vi "Voltage - Continuous Input.vi"() -> ()   [LabVIEW 2018]
doc: "This example demonstrates how to continuously acquire buffered voltage measurements using a DAQmx device.\n\nFor instructions on how to connect your signals to the DAQ device, refer to your device documentation."
uses:
  <vilib>/DAQmx/read.llb/DAQmx Read (Analog 1D Wfm NChan NSamp).vi
  <vilib>/DAQmx/create/channels.llb/DAQmx Create Channel (AI-Voltage-Basic).vi
  <vilib>/DAQmx/configure/timing.llb/DAQmx Timing (Sample Clock).vi
  <vilib>/DAQmx/configure/task.llb/DAQmx Configure Logging (TDMS).vi
  <vilib>/DAQmx/configure/trigger.llb/DAQmx Start Trigger (Digital Edge).vi
  <vilib>/DAQmx/miscellaneous.llb/DAQmx Fill In Error Info.vi
  <resource>/objmgr/daqmx.rc
panel:
  in  "edge 2":i32(ring)=10280 items=["Rising"=10280, "Falling"=10171]
  in  "source 2":tag
  in  "Stop":bool
  out "Waveform Graph":waveform(dbl)[](graph)
  in  "TDMS File Path":path
  in  "Samples per Loop":i32=1000
  in  "Sample Rate":dbl=1000.0
  in  "Sample Clock Source":tag="OnboardClock"
  in  "Terminal Configuration":i32(ring)=-1 items=["default"=-1, "RSE"=10083, "NRSE"=10078, "Differential"=10106, "Pseudodifferential"=12529]
  in  "Max Voltage":dbl=5.0
  in  "Min Voltage":dbl=-5.0
  in  "Physical Channel":tag="Dev1/ai0"
  out "Actual Sample Rate":dbl=1000.0 format="%0.2f"
  in  "Logging Mode":i32(ring)=10231 items=["Off"=10231, "Log and Read"=15842]
  # "Channel Settings"
  # "Acquired Data"
  # "Timing Settings"
  # "Logging Settings"
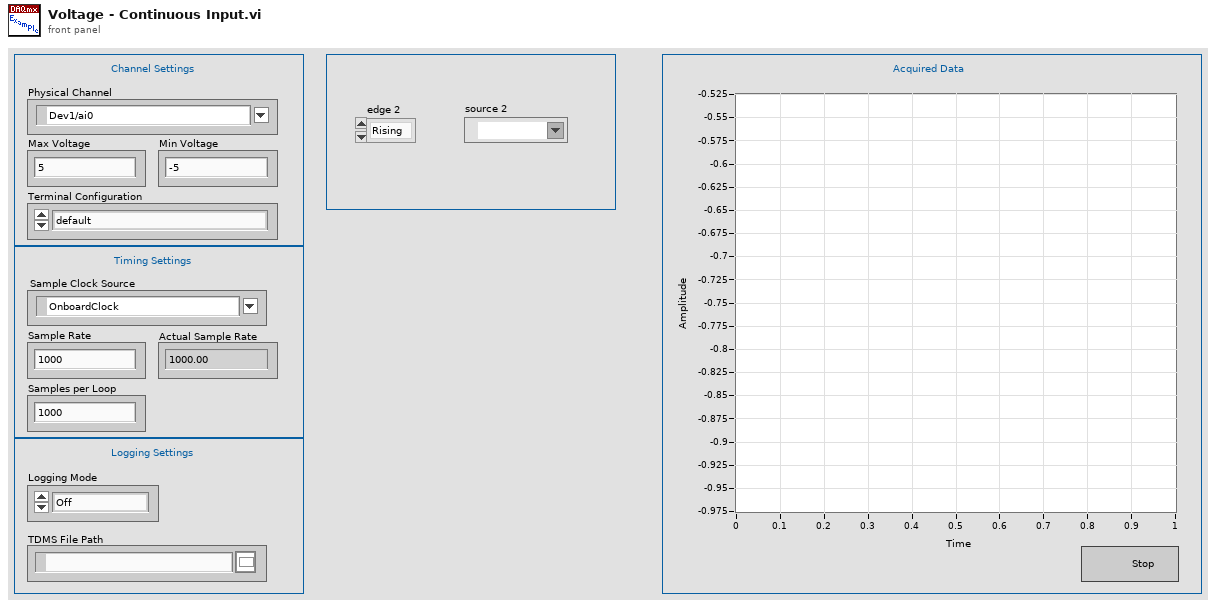
[diagram p1: front panel]
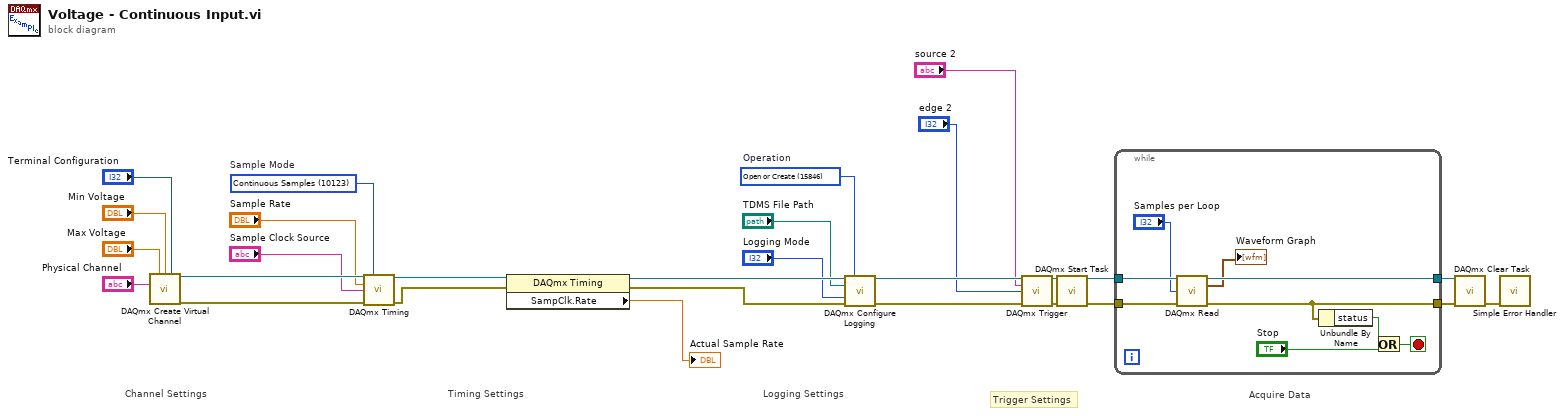
[diagram p0: block diagram]
diagram:
  w20 = 15846 items=["Open"=10437, "Open or Create"=15846, "Create or Replace"=15847, "Create"=15848]  # Operation
  w25 = 10123 items=["Finite Samples"=10178, "Continuous Samples"=10123, "Hardware Timed Single Point"=12522]  # Sample Mode
  # "Trigger Settings"
  # "Acquire Data"
  # "Timing Settings"
  # "Channel Settings"
  # "Logging Settings"
  n1 = call-poly <vilib>:"DAQmx Create Virtual Channel.vi"("maximum value"="Max Voltage", "minimum value"="Min Voltage", "input terminal configuration"="Terminal Configuration", "physical channels"="Physical Channel") -> ("task out"=w23:refnum<k21>, "error out"=w24:errorcluster)  [unwired: 10 in]
  n2 = call-poly <vilib>:"DAQmx Timing.vi"("task/channels in"=w23, "sample mode"=w25, "rate"="Sample Rate", "source"="Sample Clock Source", "error in"=w24) -> ("task out"=w27:refnum<k21>, "error out"=w26:errorcluster)  [unwired: 9 in]
  n3 = property class="DAQmx Timing"(reference=w27, error in=w26) -> (reference out=w22:refnum<k21>, error out=w21:errorcluster, "SampClk.Rate"=→"Actual Sample Rate":dbl)
  n4 = call-poly <vilib>:"DAQmx Configure Logging.vi"("task/channels in"=w22, "operation"=w20, "file path"="TDMS File Path", "logging mode"="Logging Mode", "error in"=w21) -> ("task out"=w5:refnum<k21>, "error out"=w4:errorcluster)  [unwired: 9 in]
  n5 = call-poly <vilib>:"DAQmx Trigger.vi"("task/channels in"=w5, "source"="source 2", "edge"="edge 2") -> ("task out"=w3:refnum<k21>)  [unwired: 11 in, 1 out]
  n6 = call <vilib>:"DAQmx Start Task.vi"("task/channels in"=w3, "error in"=w4) -> ("task out"=w19:refnum<k21>, "error out"=w18:errorcluster)  [unwired: 12 in]
  n7 = while {
    tunnel: w19 -> [w36]
    tunnel: w18 -> [w35]
    tunnel: [w32] -> w16
    tunnel: [w33] -> w17
    stop <- w34 stop-if-true
    n8 = call-poly <vilib>:"DAQmx Read.vi"("task/channels in"=w36, "number of samples per channel"="Samples per Loop", "error in"=w35) -> ("task out"=w33:refnum<k21>, "data"=→"Waveform Graph":waveform(dbl)[], "error out"=w32:errorcluster)  [unwired: 10 in]
    n9 = Unbundle By Name(w32) -> ("status"=w31:bool)
    n10 = Or(x=w31, y="Stop") -> (x .or. y?=w34:bool)
  }
  n11 = call <vilib>:"DAQmx Clear Task.vi"("task in"=w17, "error in"=w16) -> ("error out"=w15:errorcluster)  [unwired: 13 in]
  n12 = call <vilib>:"Simple Error Handler.vi"("error in (no error)"=w15) -> ()  [unwired: 4 in, 5 out]
